vi "CarWashTestcase.vi"(11 "error in":errorcluster) -> (15 "error out":errorcluster)   [LabVIEW 2016, in "CarWashTest.lvlib"]
doc: "Perform test for Car Wash"
uses:
  CarWashTest.lvlib
  Controls/WashStepConfig.ctl
  <vilib>/addons/_JKI Toolkits/Caraya/classes/Test/Test.lvclass
panel:
  out "Wash Array":T1[](array[typedef])
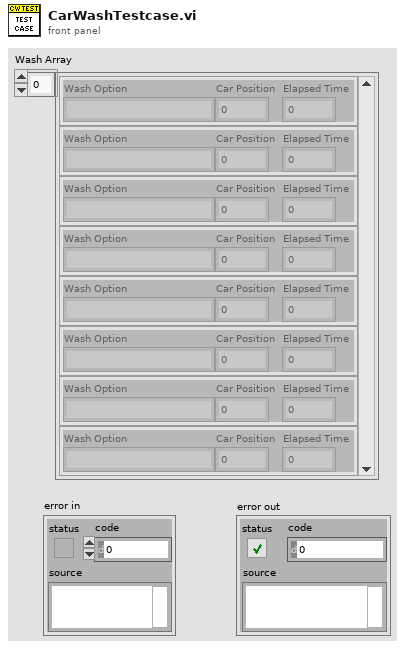
[diagram p1: front panel]
types:
  T1 = typedef "CarWashTest.lvlib/WashStepConfig.ctl" = cluster{"Wash Option":string, "Car Position":i32, "Elapsed Time":dbl}
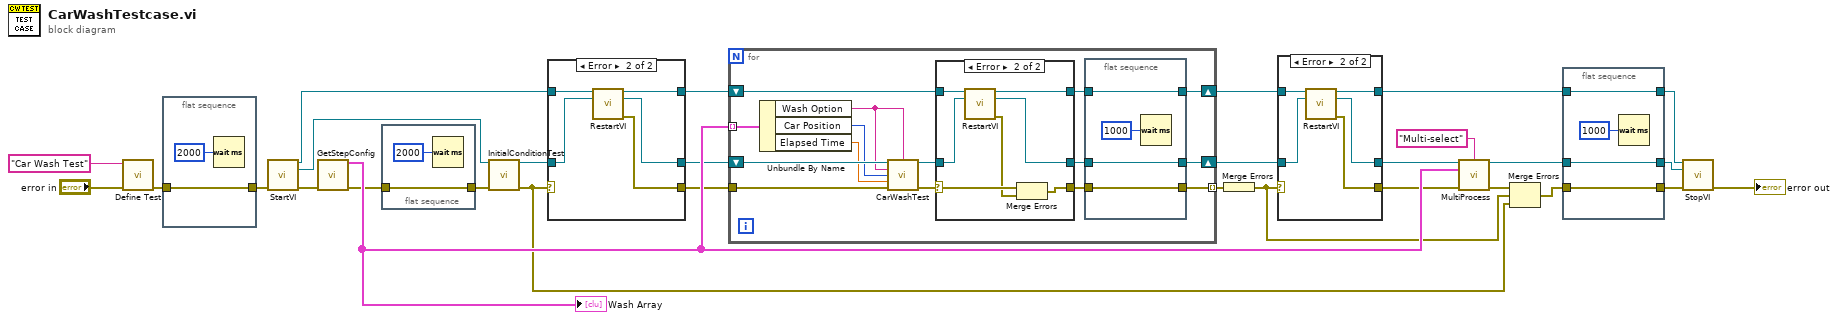
[diagram p0: block diagram]
diagram:
  n1 = call <vilib>:"Define Test.vi"("error in (no error)"="error in", "Label (VI Title)"="Car Wash Test" ("Label")) -> ("error out"=w12:errorcluster)  [unwired: 8 in, 1 out]
  n2 = flat-sequence {
    tunnel: [w31] -> w27
    tunnel: w12 -> [w31]
    frame #0 {
      n3 = Wait (ms)(milliseconds to wait=u32 2000) -> ()  [unwired: 1 out]
    }
  }
  n4 = call "StartVI.vi"("error in"=w27) -> ("Application Ref out"=w28:refnum<vi>, "VI Reference"=w29:refnum<vi>, "error out"=w30:errorcluster)  [unwired: 12 in]
  n5 = call "GetStepConfig.vi"("error in"=w30) -> ("Wash Array"=w26:T1[], "error out"=w2:errorcluster)  [unwired: 13 in]
  "Wash Array" <- w26
  n6 = flat-sequence {
    tunnel: [w33] -> w1
    tunnel: w2 -> [w33]
    frame #0 {
      n7 = Wait (ms)(milliseconds to wait=u32 2000) -> ()  [unwired: 1 out]
    }
  }
  n8 = call "InitialConditionTest.vi"("VI Reference In"=w29, "error in"=w1) -> ("VI Reference Out"=w19:refnum<vi>, "error out"=w22:errorcluster)  [unwired: 12 in]
  n9 = case shown="Error" w22 {
    selector: w22 -> [w36 _]
    tunnel: [w36 w42] -> w25
    tunnel: w19 -> [w37 w40]
    tunnel: [w37 w41] -> w20
    tunnel: [w35 w38] -> w18
    tunnel: w28 -> [w35 w39]
    frame No Error {
    }
    frame Error {
      n10 = call "RestartVI.vi"("Application Ref in"=w39, "VI in"=w40) -> ("Application Ref out"=w38:refnum<vi>, "VI out"=w41:refnum<vi>, "error out"=w42:errorcluster)  [unwired: 11 in]
    }
  }
  n11 = for {
    shift-right: [w46] -> w14
    shift-left: w20 -> [w56]
    tunnel: w26 -> [w55] mode=indexing
    tunnel: w25 -> [w57]
    tunnel: [w49] -> w7 mode=indexing
    shift-right: [w45] -> w13
    shift-left: w18 -> [w43]
    n12 = Unbundle By Name(w55) -> ("Wash Option"=w52:string, "Car Position"=w54:i32, "Elapsed Time"=w53:dbl)
    n13 = call "CarWashTest.vi"("VI Reference In"=w56, "Label"=w52, "Wash Option"=w52, "Car Position"=w54, "Elapsed Time"=w53, "error in"=w57) -> ("VI Reference Out"=w50:refnum<vi>, "error out"=w51:errorcluster)  [unwired: 8 in]
    n14 = case shown="Error" w51 {
      selector: w51 -> [w63 w71]
      tunnel: [w63 w70] -> w48
      tunnel: w50 -> [w64 w68]
      tunnel: [w64 w65] -> w47
      tunnel: [w62 w66] -> w44
      tunnel: w43 -> [w62 w67]
      frame No Error {
      }
      frame Error {
        n15 = call "RestartVI.vi"("Application Ref in"=w67, "VI in"=w68) -> ("Application Ref out"=w66:refnum<vi>, "VI out"=w65:refnum<vi>, "error out"=w69:errorcluster)  [unwired: 11 in]
        n16 = Merge Errors(w71, w69) -> (w70:errorcluster)
      }
    }
    n17 = flat-sequence {
      tunnel: [w61] -> w49
      tunnel: w48 -> [w61]
      tunnel: w47 -> [w60]
      tunnel: [w60] -> w46
      tunnel: [w59] -> w45
      tunnel: w44 -> [w59]
      frame #0 {
        n18 = Wait (ms)(milliseconds to wait=u32 1000) -> ()  [unwired: 1 out]
      }
    }
  }
  n19 = Merge Errors(w7) -> (w23:errorcluster)
  n20 = case shown="Error" w23 {
    selector: w23 -> [w73 _]
    tunnel: [w73 w79] -> w17
    tunnel: w14 -> [w74 w77]
    tunnel: [w74 w78] -> w15
    tunnel: [w72 w75] -> w16
    tunnel: w13 -> [w72 w76]
    frame No Error {
    }
    frame Error {
      n21 = call "RestartVI.vi"("Application Ref in"=w76, "VI in"=w77) -> ("Application Ref out"=w75:refnum<vi>, "VI out"=w78:refnum<vi>, "error out"=w79:errorcluster)  [unwired: 11 in]
    }
  }
  n22 = call "MultiProcess.vi"("VI Reference In"=w15, "Label"="Multi-select", "Wash Array"=w26, "error in"=w17) -> ("VI Reference Out"=w8:refnum<vi>, "error out"=w24:errorcluster)  [unwired: 10 in]
  n23 = Merge Errors(w24, w23, w22) -> (w21:errorcluster)
  n24 = flat-sequence {
    tunnel: [w83] -> w11
    tunnel: w21 -> [w83]
    tunnel: w8 -> [w80]
    tunnel: [w82] -> w10
    tunnel: w16 -> [w82]
    tunnel: [w80] -> w9
    frame #0 {
      n25 = Wait (ms)(milliseconds to wait=u32 1000) -> ()  [unwired: 1 out]
    }
  }
  n26 = call "StopVI.vi"("Application Ref in"=w10, "VI in"=w9, "error in (no error)"=w11) -> ("error out"=→"error out":errorcluster)  [unwired: 12 in]
